vi "LINC Config Global.vi"(5 "target name":string, 7 "mode":T2, 8 "error in (no error)":errorcluster, 10 "config in":T1) -> (0 "error out":errorcluster, 2 "config out":T1)   [LabVIEW 2018, in "STEPkgDriver_LINC.lvlib"]
uses:
  STEPkgDriver_LINC.lvlib
  LINC Config.ctl
  LINC Global Config Mode.ctl
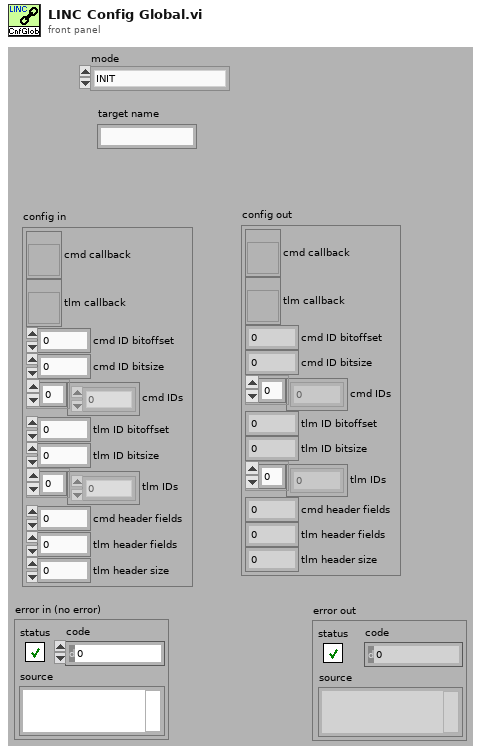
[diagram p1: front panel]
types:
  T1 = typedef "STEPkgDriver_LINC.lvlib/LINC Config.ctl" = cluster{"cmd callback":refnum<vi>, "tlm callback":refnum<vi>, "cmd ID bitoffset":i32, "cmd ID bitsize":i32, "cmd IDs":i32[], "tlm ID bitoffset":i32, "tlm ID bitsize":i32, "tlm IDs":i32[], "cmd header fields":i32, "tlm header fields":i32, "tlm header size":i32}
  T2 = typedef "STEPkgDriver_LINC.lvlib/LINC Global Config Mode.ctl" = enum16{"INIT", "CLEAR", "SET_CMD_CB", "SET_TLM_CB", "SET_CMD_FIELDS", "SET_TLM_FIELDS", "SET_ID", "GET_CONFIG"}
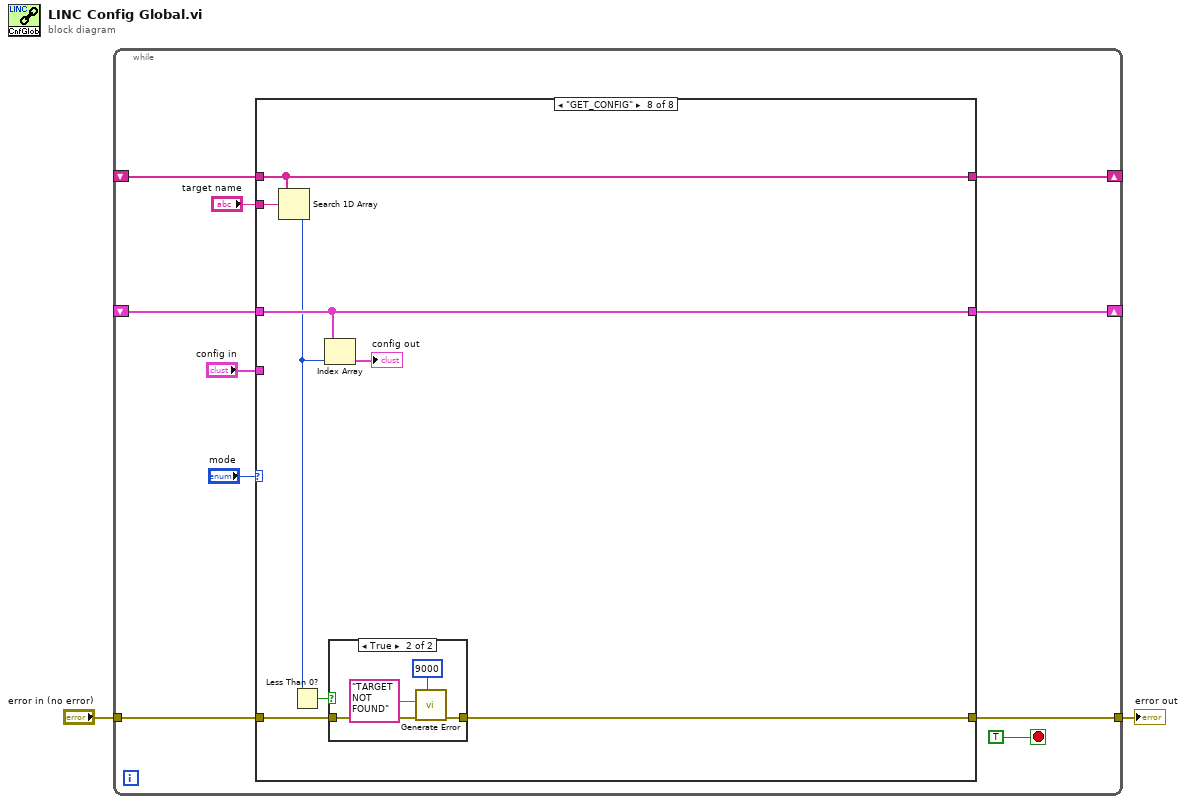
[diagram p0: block diagram]
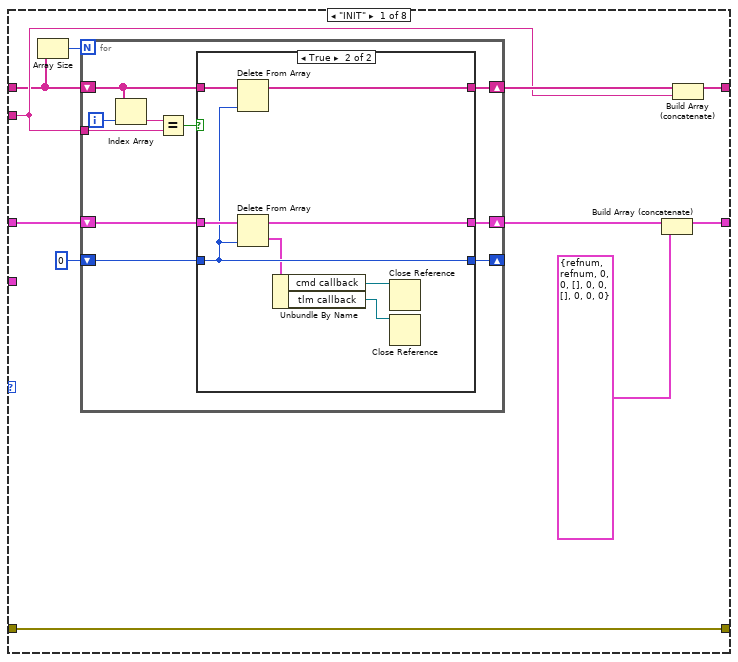
[diagram p2: hidden frame]
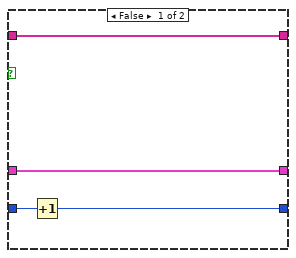
[diagram p3: hidden frame]
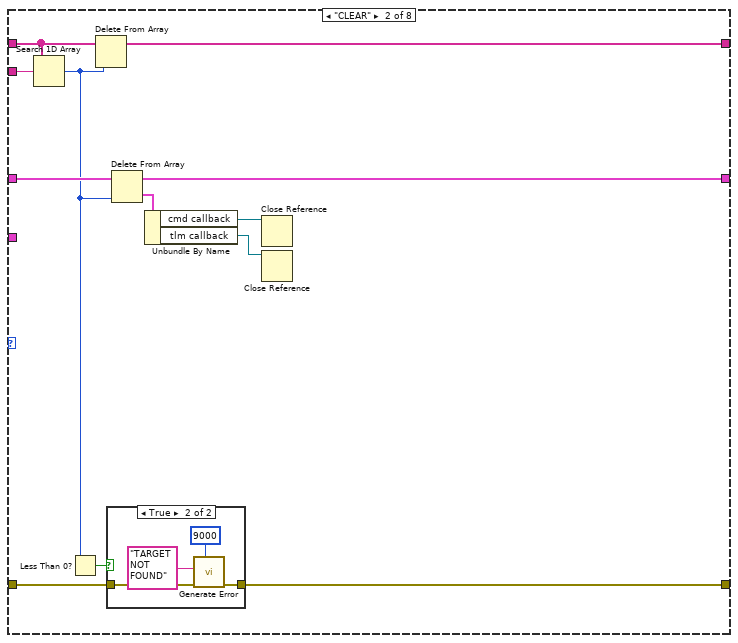
[diagram p4: hidden frame]
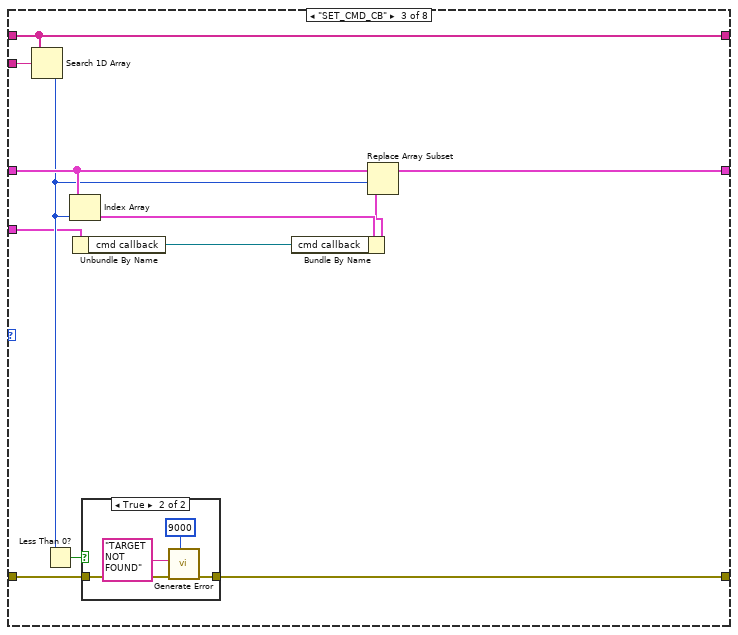
[diagram p6: hidden frame]
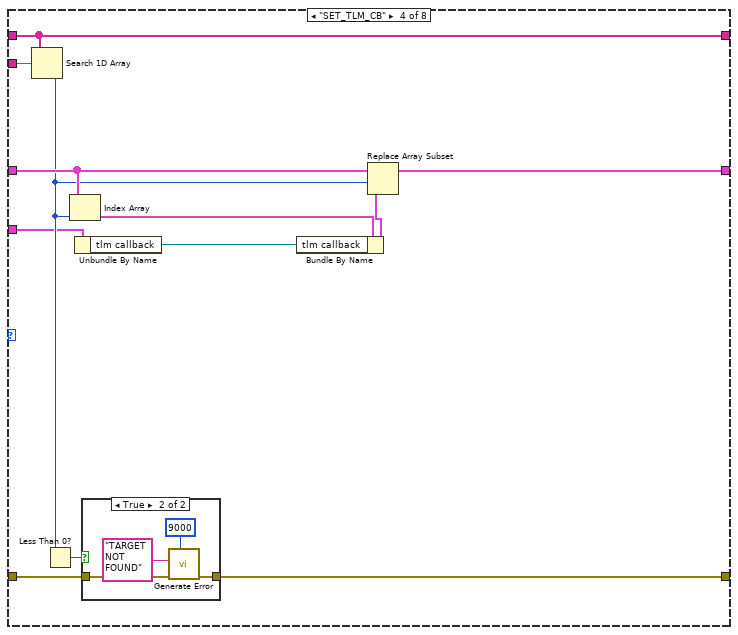
[diagram p8: hidden frame]
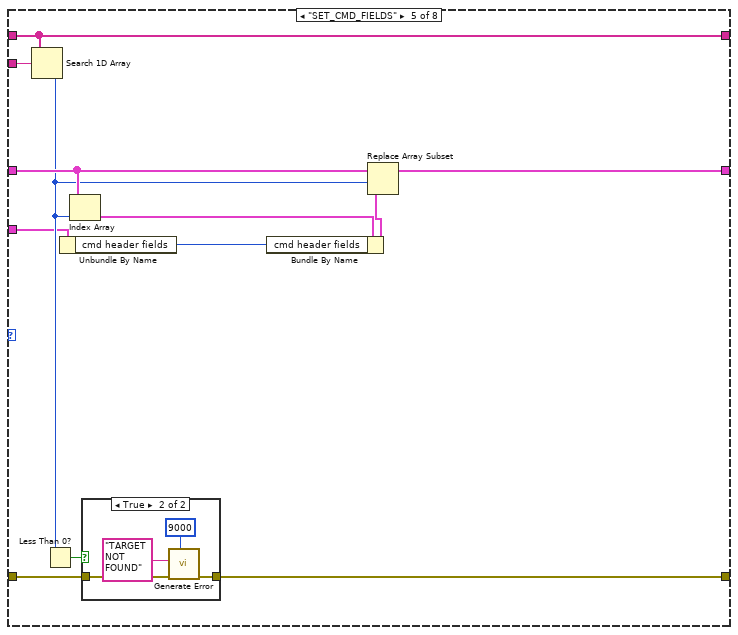
[diagram p10: hidden frame]
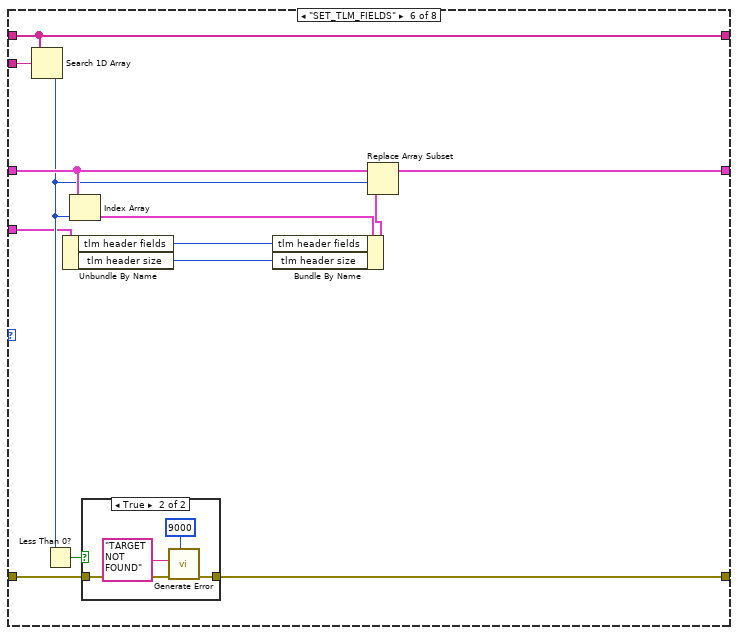
[diagram p12: hidden frame]
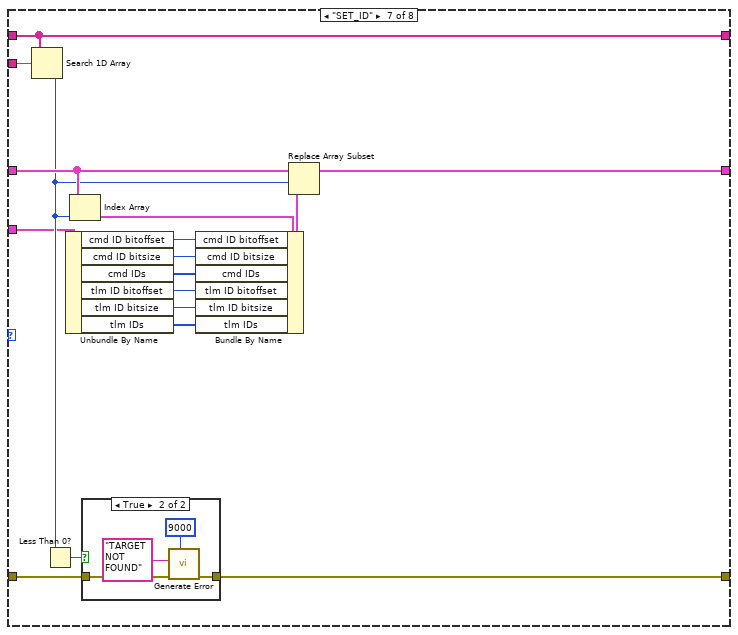
[diagram p14: hidden frame]
diagram:
  n1 = while {
    shift-right: [w10] -> _
    shift-left: _ -> [w11]
    tunnel: "error in (no error)" -> [w7]
    tunnel: [w6] -> w1
    shift-right: [w4] -> _
    shift-left: _ -> [w5]
    stop <- TRUE stop-if-true
    n2 = case shown="\"GET_CONFIG\"" "mode" {
      tunnel: w11 -> [w16 w56 w73 w90 w107 w125 w147 w160]
      tunnel: [w23 w55 w73 w90 w107 w125 w147 w160] -> w10
      tunnel: "target name" -> [w17 w57 w74 w91 w108 w126 w148 w161]
      tunnel: w7 -> [w22 w53 w70 w87 w104 w122 w145 w156]
      tunnel: [w22 w52 w69 w86 w103 w121 w144 w155] -> w6
      tunnel: w5 -> [w18 w51 w68 w85 w102 w120 w141 w159]
      tunnel: [w20 w50 w72 w89 w106 w124 w140 w159] -> w4
      tunnel: "config in" -> [_ _ w64 w81 w98 w116 w138 _]
      frame "INIT" {
        n3 = Array Size(array=w16) -> (size(s)=w15:i32)
        n4 = for {
          N: w15 -> [_]
          shift-right: [w27] -> w19
          shift-left: w16 -> [w32]
          shift-right: [w26] -> w13
          shift-left: w18 -> [w31]
          tunnel: w17 -> [w29]
          shift-right: [w24] -> _
          shift-left: 0 -> [w25]
          i -> [w33]
          n5 = Index Array(array=w32, index=w33) -> (element=w30:string)
          n6 = Equal?(x=w30, y=w29) -> (x = y?=w28:bool)
          n7 = case shown="True" w28 {
            tunnel: w32 -> [w37 w45]
            tunnel: w31 -> [w36 w43]
            tunnel: [w37 w44] -> w27
            tunnel: [w36 w42] -> w26
            tunnel: w25 -> [w35 w41]
            tunnel: [w34 w41] -> w24
            frame False {
              n8 = Increment(x=w35) -> (x+1=w34:i32)
            }
            frame True {
              n9 = Delete From Array(array=w45, index=w41) -> (array with subset deleted=w44:string[])  [unwired: 1 in, 1 out]
              n10 = Delete From Array(array=w43, index=w41) -> (deleted portion=w38:T1, array with subset deleted=w42:T1[])  [unwired: 1 in]
              n11 = Unbundle By Name(w38) -> ("cmd callback"=w40:refnum<vi>, "tlm callback"=w39:refnum<vi>)
              n12 = Close Reference(reference=w40) -> ()  [unwired: 1 in, 1 out]
              n13 = Close Reference(reference=w39) -> ()  [unwired: 1 in, 1 out]
            }
          }
        }
        n14 = Build Array (concatenate)(w13, T1 {"cmd callback"=refnum, "tlm callback"=refnum, "cmd ID bitoffset"=0, "cmd ID bitsize"=0, "cmd IDs"=[], "tlm ID bitoffset"=0, "tlm ID bitsize"=0, "tlm IDs"=[], "cmd header fields"=0, "tlm header fields"=0, "tlm header size"=0} ("housekeeping in")) -> (w20:T1[])
        n15 = Build Array (concatenate)(w19, w17) -> (w23:string[])
      }
      frame "CLEAR" {
        n16 = Search 1D Array(1D array=w56, element=w57) -> (index of element=w49:i32)  [unwired: 1 in]
        n17 = Less Than 0?(x=w49) -> (x < 0?=w54:bool)
        n18 = Delete From Array(array=w56, index=w49) -> (array with subset deleted=w55:string[])  [unwired: 1 in, 1 out]
        n19 = case shown="True" w54 {
          tunnel: w53 -> [w58 w62]
          tunnel: [w58 w61] -> w52
          frame False {
          }
          frame True {
            n20 = call "Generate Error.vi"("error code (-1301)"=9000, "error in"=w62, "description"="TARGET NOT FOUND") -> ("error out"=w61:errorcluster)  [unwired: 8 in]
          }
        }
        n21 = Delete From Array(array=w51, index=w49) -> (deleted portion=w48:T1, array with subset deleted=w50:T1[])  [unwired: 1 in]
        n22 = Unbundle By Name(w48) -> ("cmd callback"=w47:refnum<vi>, "tlm callback"=w46:refnum<vi>)
        n23 = Close Reference(reference=w47) -> ()  [unwired: 1 in, 1 out]
        n24 = Close Reference(reference=w46) -> ()  [unwired: 1 in, 1 out]
      }
      frame "SET_CMD_CB" {
        n25 = Search 1D Array(1D array=w73, element=w74) -> (index of element=w67:i32)  [unwired: 1 in]
        n26 = Less Than 0?(x=w67) -> (x < 0?=w71:bool)
        n27 = Index Array(array=w68, index=w67) -> (element=w66:T1)
        n28 = Unbundle By Name(w64) -> ("cmd callback"=w63:refnum<vi>)
        n29 = case shown="True" w71 {
          tunnel: w70 -> [w75 w79]
          tunnel: [w75 w78] -> w69
          frame False {
          }
          frame True {
            n30 = call "Generate Error.vi"("error code (-1301)"=9000, "error in"=w79, "description"="TARGET NOT FOUND") -> ("error out"=w78:errorcluster)  [unwired: 8 in]
          }
        }
        n31 = Bundle By Name(cluster=w66, "cmd callback"=w63) -> (w65:T1)
        n32 = Replace Array Subset(array=w68, new element=w65, index=w67) -> (w72:T1[])
      }
      frame "SET_TLM_CB" {
        n33 = Search 1D Array(1D array=w90, element=w91) -> (index of element=w84:i32)  [unwired: 1 in]
        n34 = Less Than 0?(x=w84) -> (x < 0?=w88:bool)
        n35 = Index Array(array=w85, index=w84) -> (element=w83:T1)
        n36 = Unbundle By Name(w81) -> ("tlm callback"=w80:refnum<vi>)
        n37 = case shown="True" w88 {
          tunnel: w87 -> [w92 w96]
          tunnel: [w92 w95] -> w86
          frame False {
          }
          frame True {
            n38 = call "Generate Error.vi"("error code (-1301)"=9000, "error in"=w96, "description"="TARGET NOT FOUND") -> ("error out"=w95:errorcluster)  [unwired: 8 in]
          }
        }
        n39 = Bundle By Name(cluster=w83, "tlm callback"=w80) -> (w82:T1)
        n40 = Replace Array Subset(array=w85, new element=w82, index=w84) -> (w89:T1[])
      }
      frame "SET_CMD_FIELDS" {
        n41 = Search 1D Array(1D array=w107, element=w108) -> (index of element=w101:i32)  [unwired: 1 in]
        n42 = Less Than 0?(x=w101) -> (x < 0?=w105:bool)
        n43 = Unbundle By Name(w98) -> ("cmd header fields"=w97:i32)
        n44 = Index Array(array=w102, index=w101) -> (element=w100:T1)
        n45 = case shown="True" w105 {
          tunnel: w104 -> [w109 w113]
          tunnel: [w109 w112] -> w103
          frame False {
          }
          frame True {
            n46 = call "Generate Error.vi"("error code (-1301)"=9000, "error in"=w113, "description"="TARGET NOT FOUND") -> ("error out"=w112:errorcluster)  [unwired: 8 in]
          }
        }
        n47 = Bundle By Name(cluster=w100, "cmd header fields"=w97) -> (w99:T1)
        n48 = Replace Array Subset(array=w102, new element=w99, index=w101) -> (w106:T1[])
      }
      frame "SET_TLM_FIELDS" {
        n49 = Search 1D Array(1D array=w125, element=w126) -> (index of element=w119:i32)  [unwired: 1 in]
        n50 = Less Than 0?(x=w119) -> (x < 0?=w123:bool)
        n51 = Unbundle By Name(w116) -> ("tlm header fields"=w115:i32, "tlm header size"=w114:i32)
        n52 = Index Array(array=w120, index=w119) -> (element=w118:T1)
        n53 = case shown="True" w123 {
          tunnel: w122 -> [w127 w131]
          tunnel: [w127 w130] -> w121
          frame False {
          }
          frame True {
            n54 = call "Generate Error.vi"("error code (-1301)"=9000, "error in"=w131, "description"="TARGET NOT FOUND") -> ("error out"=w130:errorcluster)  [unwired: 8 in]
          }
        }
        n55 = Bundle By Name(cluster=w118, "tlm header fields"=w115, "tlm header size"=w114) -> (w117:T1)
        n56 = Replace Array Subset(array=w120, new element=w117, index=w119) -> (w124:T1[])
      }
      frame "SET_ID" {
        n57 = Search 1D Array(1D array=w147, element=w148) -> (index of element=w139:i32)  [unwired: 1 in]
        n58 = Less Than 0?(x=w139) -> (x < 0?=w146:bool)
        n59 = Unbundle By Name(w138) -> ("cmd ID bitoffset"=w137:i32, "cmd ID bitsize"=w136:i32, "cmd IDs"=w135:i32[], "tlm ID bitoffset"=w134:i32, "tlm ID bitsize"=w133:i32, "tlm IDs"=w132:i32[])
        n60 = Index Array(array=w141, index=w139) -> (element=w143:T1)
        n61 = case shown="True" w146 {
          tunnel: w145 -> [w149 w153]
          tunnel: [w149 w152] -> w144
          frame False {
          }
          frame True {
            n62 = call "Generate Error.vi"("error code (-1301)"=9000, "error in"=w153, "description"="TARGET NOT FOUND") -> ("error out"=w152:errorcluster)  [unwired: 8 in]
          }
        }
        n63 = Bundle By Name(cluster=w143, "cmd ID bitoffset"=w137, "cmd ID bitsize"=w136, "cmd IDs"=w135, "tlm ID bitoffset"=w134, "tlm ID bitsize"=w133, "tlm IDs"=w132) -> (w142:T1)
        n64 = Replace Array Subset(array=w141, new element=w142, index=w139) -> (w140:T1[])
      }
      frame "GET_CONFIG" {
        n65 = Search 1D Array(1D array=w160, element=w161) -> (index of element=w154:i32)  [unwired: 1 in]
        n66 = Less Than 0?(x=w154) -> (x < 0?=w157:bool)
        n67 = Index Array(array=w159, index=w154) -> (element=→"config out":T1)
        n68 = case shown="True" w157 {
          tunnel: w156 -> [w162 w166]
          tunnel: [w162 w165] -> w155
          frame False {
          }
          frame True {
            n69 = call "Generate Error.vi"("error code (-1301)"=9000, "error in"=w166, "description"="TARGET NOT FOUND") -> ("error out"=w165:errorcluster)  [unwired: 8 in]
          }
        }
      }
    }
  }
  "error out" <- w1
